vi "Start Vision.vi"(8 "error in (no error)":errorcluster, 10 "Input":T1, 11 "Vision in":refnum<class "Vision.lvclass">) -> (0 "error out":errorcluster, 3 "Vision out":refnum<class "Vision.lvclass">)   [LabVIEW 2022 SP3]
uses:
  Vision.lvclass
  UDP Input.ctl
  Vision.lvclass/Vision.ctl
  UDP Data Receiver/UDP Data Receiver Messages/Start Vision Msg/Start Vision Msg 2.lvclass
  C:/Program Files (x86)/National Instruments/LabVIEW 2022/vi.lib/MGI/Monitored Actor/Monitored Actor/Monitored Actor/Monitored Actor.lvclass
  C:/Program Files (x86)/National Instruments/LabVIEW 2022/vi.lib/ActorFramework/Actor/Actor.lvclass
  C:/Users/ebert/Documents/codes/ssl/repo/Phoenix Reborn/Vision/Vision/Vision.lvclass
  C:/Users/ebert/Documents/codes/ssl/repo/Phoenix Reborn/UDP Data Receiver/UDP Data Receiver/UDP Data Receiver.lvclass
  <vilib>/ActorFramework/Message Enqueuer/Message Enqueuer.lvclass
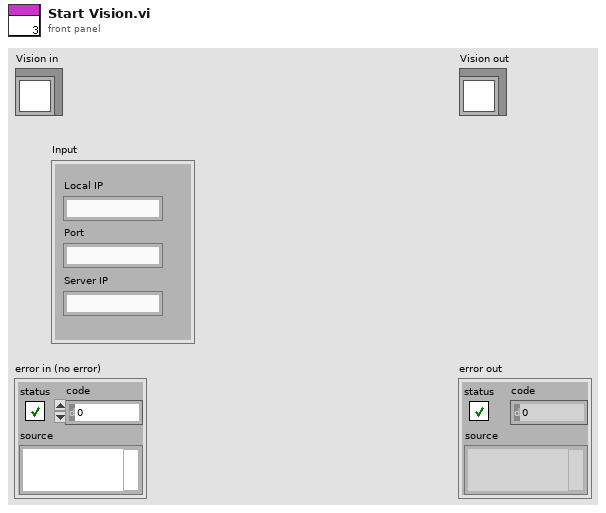
[diagram p1: front panel]
types:
  T1 = typedef "UDP Input.ctl" = cluster{"Local IP":string, "Port":string, "Server IP":string}
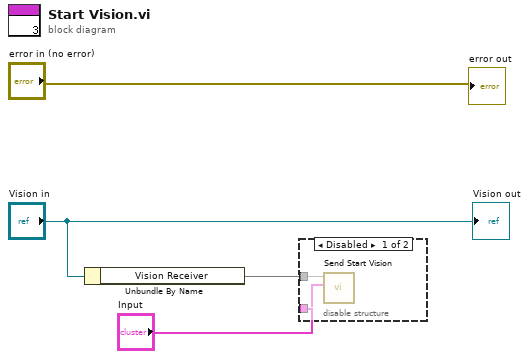
[diagram p0: block diagram]
diagram:
  n1 = Unbundle By Name("Vision in") -> ("Vision Receiver"=w3)
  n2 = disable-structure shown="Disabled" {
    disable-tunnel: w3 -> [w6 _]
    disable-tunnel: "Input" -> [w5 _]
    frame Disabled {
      n3 = call "Send Start Vision.vi"("Input"=w5, "Message Enqueuer"=w6) -> ()  [unwired: 8 in, 2 out]
    }
    frame Enabled {
    }
  }
  "error out" <- "error in (no error)"
  "Vision out" <- "Vision in"
